vi "AddCrates2.vi"(9 "To":i32, 10 "CratesToAdd":string[](array[string]), 11 "StacksIn":cluster{"Crates":string[]}[](array[cluster])) -> (3 "StacksOut":cluster{"Crates":string[]}[](array[cluster]))   [LabVIEW 2020, in "2022_5.lvclass"]
uses:
  2022_5.lvclass
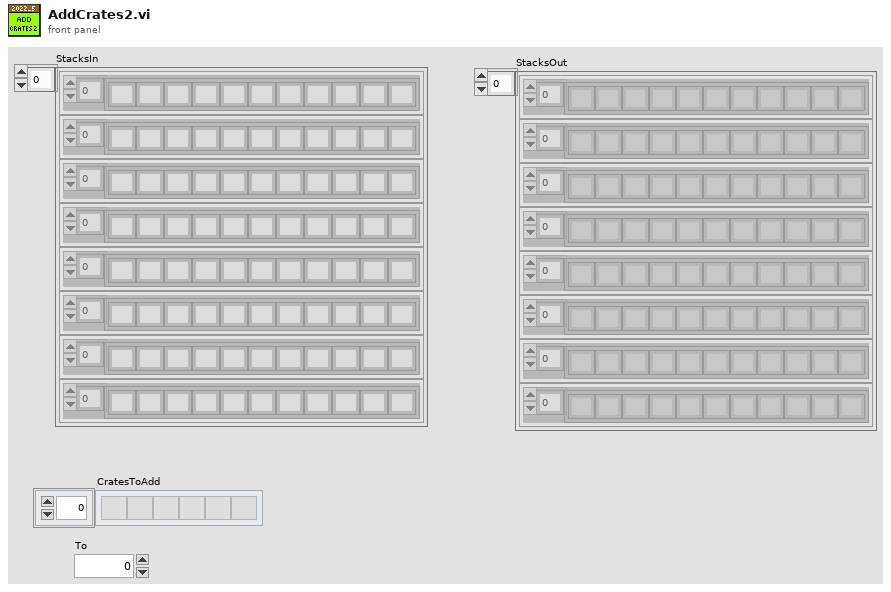
[diagram p1: front panel]
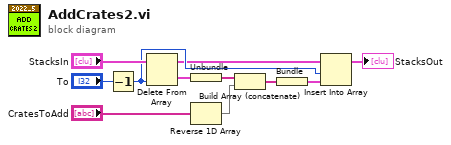
[diagram p0: block diagram]
diagram:
  n1 = Decrement(x="To") -> (x-1=w8:i32)
  n2 = Delete From Array(array="StacksIn", index=w8) -> (deleted portion=w2:cluster{"Crates":string[]}, array with subset deleted=w7:cluster{"Crates":string[]}[])  [unwired: 1 in]
  n3 = Unbundle(w2) -> ("Crates"=w6:string[])
  n4 = Reverse 1D Array(array="CratesToAdd") -> (reversed array=w4:string[])
  n5 = Build Array (concatenate)(w6, w4) -> (w3:string[])
  n6 = Bundle(w3) -> (w1:cluster{string[]})  [unwired: 1 in]
  n7 = Insert Into Array(array=w7, index=w8, new element=w1) -> (→"StacksOut":cluster{"Crates":string[]}[])
